vi "Initialise Textures.vi"(8 "error in (no error)":errorcluster, 10 "Renderer":u32, 11 "Galaxy in":refnum<class "Galaxy.lvclass">) -> (0 "error out":errorcluster, 3 "Galaxy out":refnum<class "Galaxy.lvclass">)   [LabVIEW 2021, in "Galaxy.lvclass"]
uses:
  Galaxy.lvclass
  Galaxy.lvclass/Galaxy.ctl
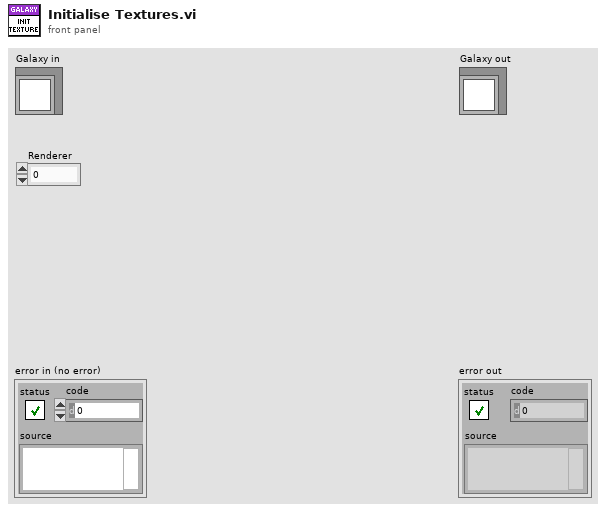
[diagram p1: front panel]
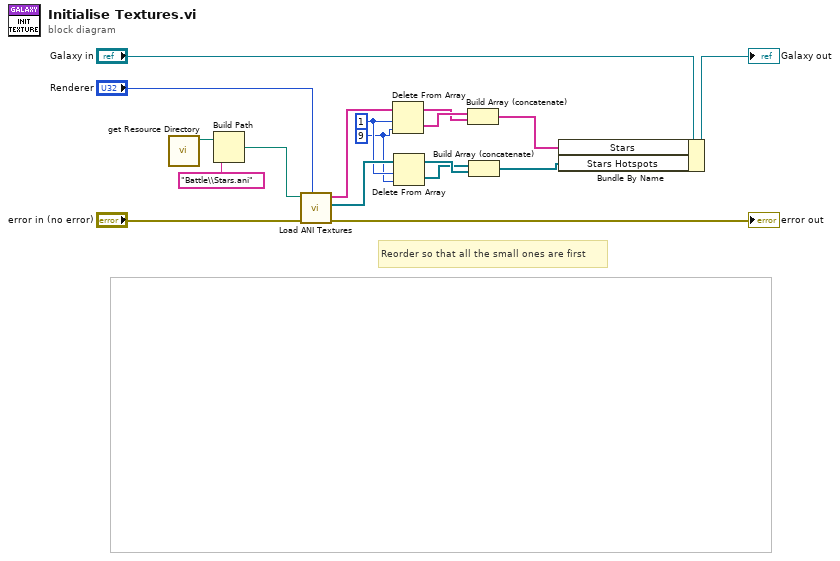
[diagram p0: block diagram]
diagram:
  w2 = 9 ("index")
  w3 = 1 ("length")
  # "Reorder so that all the small ones are first"
  n1 = call "get Resource Directory.vi"() -> ("Resource Directory"=w17:path)  [unwired: 11 in]
  n2 = Build Path(base path=w17, name or relative path="Battle\\Stars.ani") -> (appended path=w16:path)
  n3 = call "Load ANI Textures.vi"("Renderer"="Renderer", "error in (no error)"="error in (no error)", "Path"=w16) -> ("error out"=→"error out":errorcluster, "Hotspots"=w4:refnum<class "Vector 2D.lvclass">[], "Names"=w10:string[])  [unwired: 6 in]
  n4 = Delete From Array(array=w10, length=w3, index=w2) -> (deleted portion=w9:string[], array with subset deleted=w8:string[])
  n5 = Delete From Array(array=w4, length=w3, index=w2) -> (deleted portion=w5:refnum<class "Vector 2D.lvclass">[], array with subset deleted=w6:refnum<class "Vector 2D.lvclass">[])
  n6 = Build Array (concatenate)(w9, w8) -> (w7:string[])
  n7 = Build Array (concatenate)(w5, w6) -> (w1:refnum<class "Vector 2D.lvclass">[])
  n8 = Bundle By Name(cluster="Galaxy in", "Stars"=w7, "Stars Hotspots"=w1) -> (→"Galaxy out":refnum<class "Galaxy.lvclass">)
